vi "extended_uncertainty.vi"(2 "kc":dbl, 3 "Uncertainty point-by-point":dbl[](array[numeric])) -> (0 "Extended Uncertainty":dbl, 1 "Uncertainty":dbl)   [LabVIEW 2021, in "CALIBRATION.lvlib"]
uses:
  CALIBRATION.lvlib
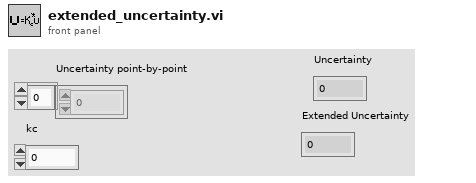
[diagram p1: front panel]
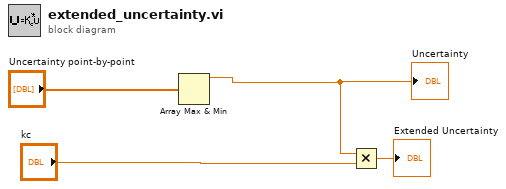
[diagram p0: block diagram]
diagram:
  n1 = Array Max & Min(array="Uncertainty point-by-point") -> (max value=w1:dbl)  [unwired: 3 out]
  "Uncertainty" <- w1
  n2 = Multiply(x=w1, y="kc") -> (x*y=→"Extended Uncertainty":dbl)
